vi "RT Main.vi"() -> ()   [LabVIEW 2014]
uses:
  SubVIs/myRIO/Controls/Switch Schedule.ctl
  SubVIs/myRIO/Controls/Switch Program.ctl
  SubVIs/myRIO/Controls/Action Enum.ctl
  SubVIs/myRIO/Controls/Switch Day.ctl
  SubVIs/myRIO/Controls/Switch Schedule FGV.ctl
  SubVIs/myRIO/Controls/myRIO Data.ctl
panel:
  in  "Host IP":string="172.22.11.1"
  out "current time":timestamp=timestamp(3481034400 s since 1904-01-01)
  in  "Switch Schedule":T1
  out "Incoming Message":string
  in  "stop":bool
  # "Smartphone Instructions\n1.  Set up your myRIO for WiFi.\n2.  Install a UDP app for your\n     smartphone.\n3.  Run RT Main.vi.\n3.  Enter the myRIO's IP address\n    into the app.\n4. Send \"on\" or \"off\"\n5. See documentation for more\n    commands."
  # "Note on Computer Control \nIf you are connected to the \nmyRIO via USB, use the virtual IP\nas shown in ipconfig.\n\nAccess ipconfig via the Start Menu.\nClick Run... and type \"cmd\". In the\nwindow that pops up, type \"ipconfig\"."
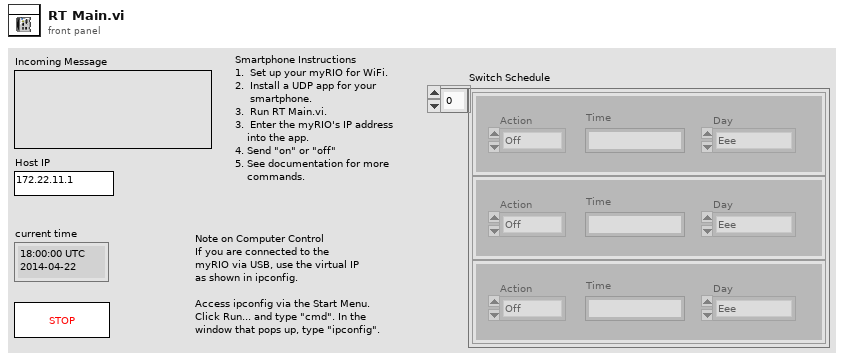
[diagram p1: front panel]
types:
  T1 = typedef "Switch Schedule.ctl" = T2[]
  T2 = typedef "Switch Program.ctl" = cluster{"Action":T3, "Time":string, "Day":T4}
  T3 = typedef "Action Enum.ctl" = enum16{"Off", "On"}
  T4 = typedef "Switch Day.ctl" = enum16{"Eee", "Sun", "Mon", "Tue", "Wed", "Thu", "Fri", "Sat"}
  T5 = typedef "Switch Schedule FGV.ctl" = enum16{"Add", "Delete", "Set", "Get", "Load", "Clear"}
  T6 = typedef "myRIO Data.ctl" = cluster{"Time":timestamp, "Switch Schedule":T1}
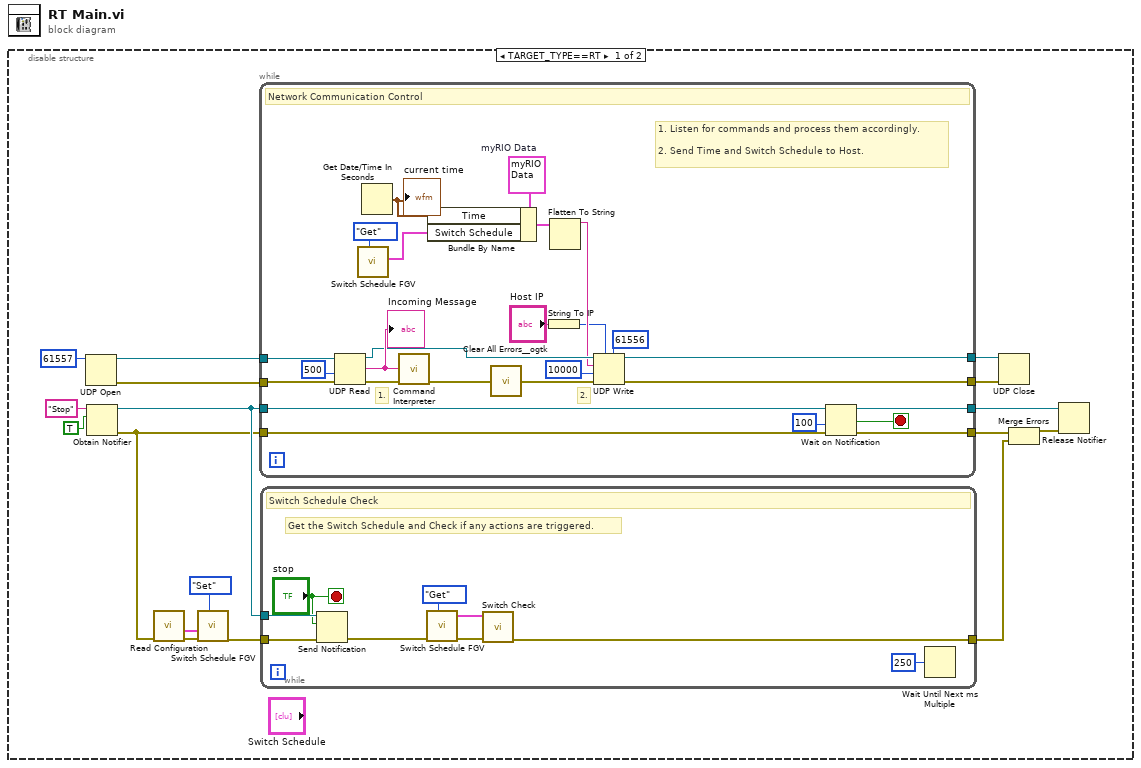
[diagram p0: block diagram]
diagram:
  n1 = disable-structure shown="TARGET_TYPE==RT" {
    frame condition #0 (active) {
      n2 = UDP Open(11:u16 61557 ("port")) -> (port=w15:refnum<k16>, 0:w16:errorcluster)  [unwired: 4 in, 1 out]
      n3 = Obtain Notifier(name (unnamed)="Stop", notification data type=TRUE ("LED0")) -> (notifier out=w10:refnum<notifier>, error out=w1:errorcluster)  [unwired: 2 in, 1 out]
      n4 = call "Read Configuration.vi"("error in (no error)"=w1) -> ("error out"=w3:errorcluster, "Switch Schedule Out"=w2:T1)  [unwired: 9 in]
      n5 = call "Switch Schedule FGV.vi"("Action"=Switch_Schedule_FGV."Set", "error in (no error)"=w3, "Switch Schedule"=w2) -> ("error out"=w4:errorcluster)  [unwired: 7 in, 1 out]
      n6 = while {
        tunnel: w16 -> [w51]
        tunnel: w15 -> [w52]
        tunnel: [w39] -> w14
        tunnel: [w38] -> w13
        tunnel: w1 -> [w48]
        tunnel: w10 -> [w49]
        tunnel: [w46] -> w9
        tunnel: [w45] -> w7
        stop <- w47 stop-if-true
        w36 = T6 {"Time"=timestamp(0 s since 1904-01-01), "Switch Schedule"=[]}  # myRIO Data
        # "2."
        # "1."
        # "1. Listen for commands and process them accordingly.\n\n2. Send Time and Switch Schedule to Host."
        # "Network Communication Control"
        n7 = UDP Read(connection ID=w52, timeout ms (25000)=500, 8:w51) -> (data out=w42:string, error out=w43:errorcluster, 3:w40:refnum<k16>)  [unwired: 1 in, 2 out]
        "Incoming Message" <- w42
        n8 = call "Switch Schedule FGV.vi"("Action"=Switch_Schedule_FGV."Get") -> ("Switch Schedule"=w34:T1)  [unwired: 9 in, 1 out]
        n9 = Get Date/Time In Seconds() -> (seconds since 1Jan1904=w35:timestamp)
        "current time" <- w35
        n10 = call "Command Interpreter.vi"("error in"=w43, "Command"=w42) -> ("error out"=w41:errorcluster)  [unwired: 9 in]
        n11 = Bundle By Name(cluster=w36, "Time"=w35, "Switch Schedule"=w34) -> (w33:T6)
        n12 = call <userlib>:"Clear All Errors__ogtk.vi"("Error In"=w41) -> ("Error Out"=w27:errorcluster)  [unwired: 3 in]
        n13 = String To IP(1:"Host IP") -> (0:w29:u32)
        n14 = Flatten To String(anything=w33) -> (data string=w32:string)  [unwired: 3 in, 2 out]
        n15 = UDP Write(address=w29, port or service name=u16 61556, connection ID=w40, data in=w32, 8:w27, 9:10000 ("timeout ms (25000)")) -> (error out=w39:errorcluster, 3:w38:refnum<k16>)
        n16 = Wait on Notification(notifier=w49, timeout in ms (-1)=100, error in (no error)=w48) -> (notifier out=w46:refnum<notifier>, notification=w47:bool, error out=w45:errorcluster)  [unwired: 1 in, 1 out]
      }
      n17 = while {
        tunnel: w10 -> [w26]
        tunnel: w4 -> [w25]
        tunnel: [w22] -> w6
        stop <- "stop" stop-if-true
        # "Get the Switch Schedule and Check if any actions are triggered."
        # "Switch Schedule Check"
        n18 = Send Notification(notification="stop", notifier=w26, error in (no error)=w25) -> (error out=w18:errorcluster)  [unwired: 1 out]
        n19 = call "Switch Schedule FGV.vi"("Action"=Switch_Schedule_FGV."Get", "error in (no error)"=w18) -> ("error out"=w19:errorcluster, "Switch Schedule"=w21:T1)  [unwired: 8 in]
        n20 = call "Switch Check.vi"("error in (no error)"=w19, "Switch Schedule"=w21) -> ("error out"=w22:errorcluster)  [unwired: 9 in]
        n21 = Wait Until Next ms Multiple(millisecond multiple=u32 250) -> ()  [unwired: 1 out]
      }
      n22 = UDP Close(connection ID=w13, 8:w14) -> ()  [unwired: 2 out]
      n23 = Merge Errors(w7, w6) -> (w8:errorcluster)
      n24 = Release Notifier(notifier=w9, error in (no error)=w8) -> ()  [unwired: 1 in, 3 out]
    }
    frame condition #1 {
    }
  }
